vi "Ref_Num_Calibrate_Short.vi"(2 "Test Failed":refnum<vi>, 3 "Calibration Short Successful":refnum<vi>, 7 "LowCapMode?":refnum<vi>, 8 "error in":errorcluster, 9 "Keystate":string, 10 "Stop Test":refnum<vi>, 11 "Calibration Test":refnum<vi>) -> (0 "error out":errorcluster)   [LabVIEW 2020]
uses:
  <vilib>/Instr/_visa.llb/GPIB Status Boolean Array.ctl
  Global 1.vi
  <vilib>/Utility/error.llb/DialogType.ctl
panel:
  in  "error in 2":errorcluster
  out "LowCapMode?":bool
  out "message":string=" INSTRUCTIONS:\r\rNormal Use:  When using subVIs that incorporate the error in/error out (or error I/O) structure, place this handler where you want to inform the user of an error, typically at the end of the I/O data path, as the last action of the program.  If the error in error? is ERROR, the handler creates a message describing the error and its source.  If the type of dialog = 1 (default), the message is displayed to the user, who can only acknowedge it.  If the type = 2, the user can acknowledge the message or abort execution; aborting a program with active I/O is not recommended.  If the type = 0, no message is displayed; this is used to process the error programmatically, and the error out cluster elements are wired to individual terminals for that reason.  \r\rOther Use:\n\r\nlocal testing.  To test the error code of a subVI or function that does not have the error I/O structure, you can wire its error code and a source string to the local error code and error source inputs.  If error in error? indicates no error and error code is not equal to 0, the local code and source are substituted for the error in values, and error? is set TRUE (ERROR)."
  out "serial poll byte (Test 2)":i16
  out "serial poll byte (Test 1)":i16
  out "ibsta":T1
  in  "Cal_Step_Delay":u16
  out "Test Count":i32
  out "Failed Test Count":i32
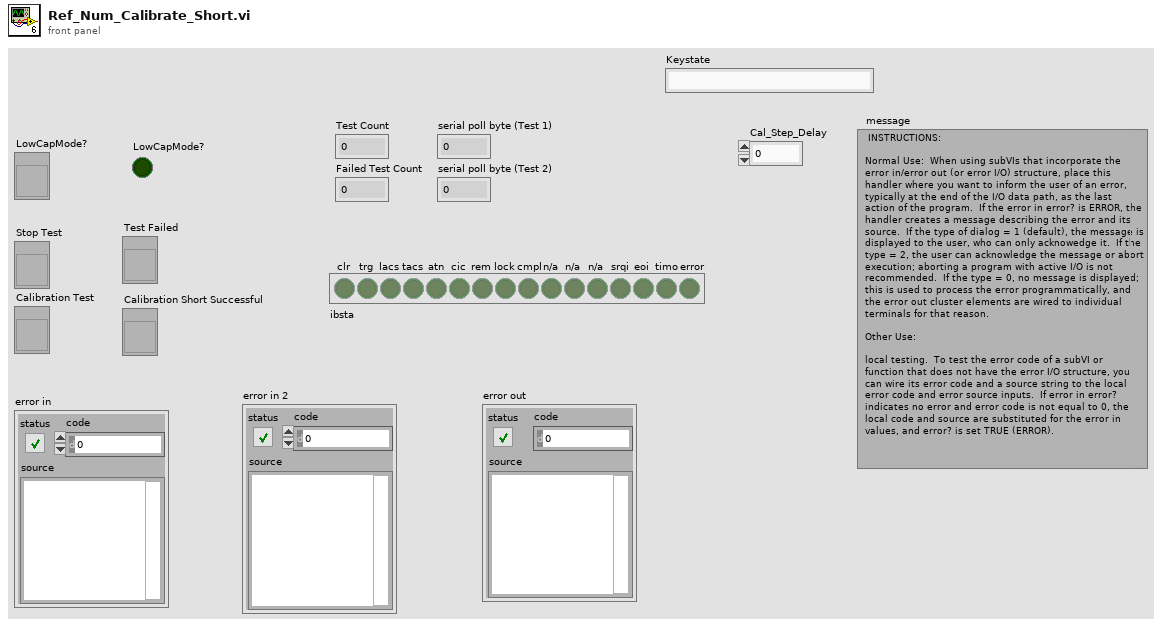
[diagram p1: front panel]
types:
  T1 = typedef "GPIB Status Boolean Array.ctl" = bool[]
  T2 = typedef "DialogType.ctl" = u16
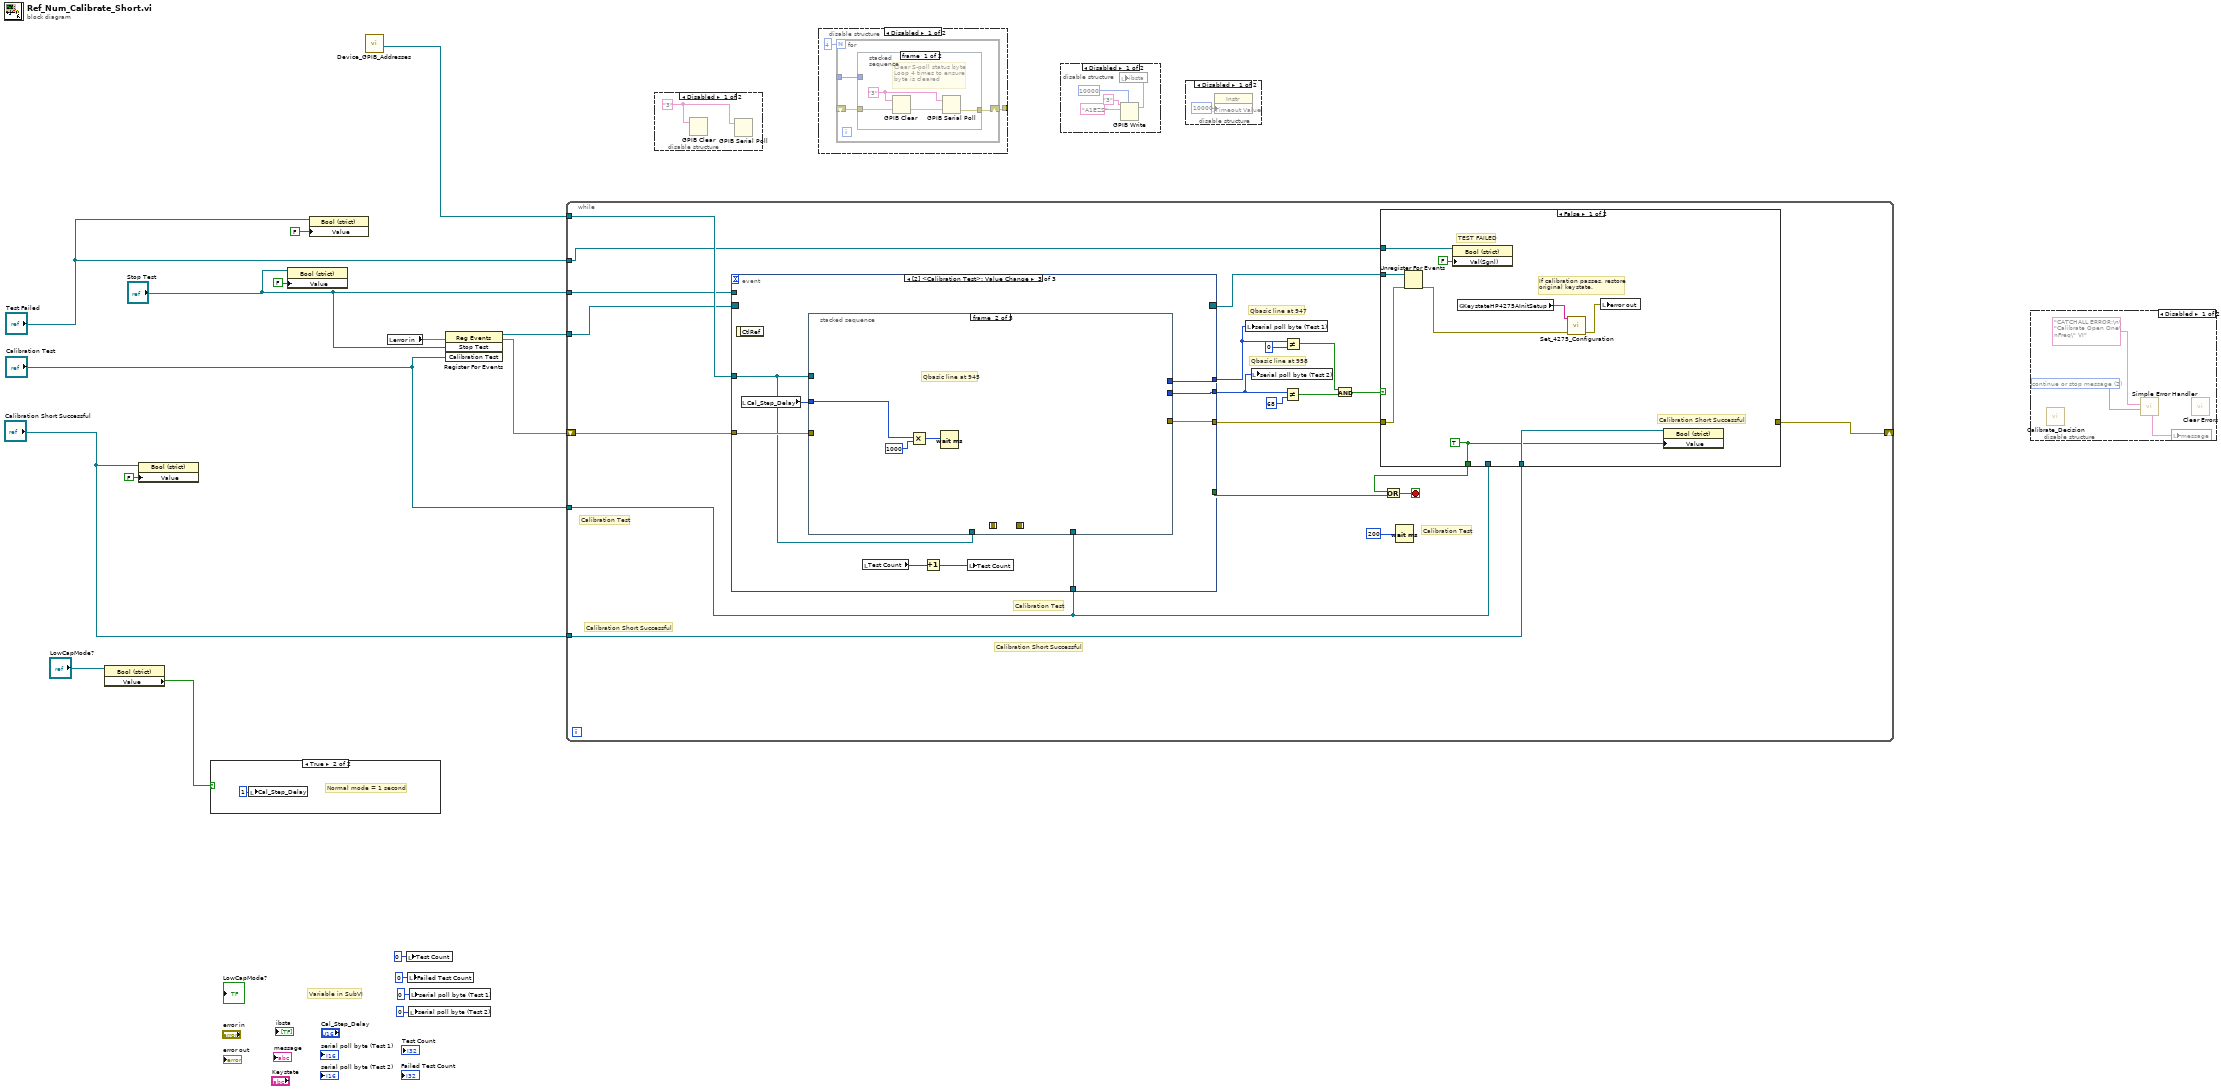
[diagram p0: block diagram]
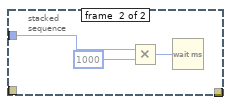
[diagram p6: hidden frame]
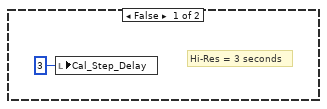
[diagram p8: hidden frame]
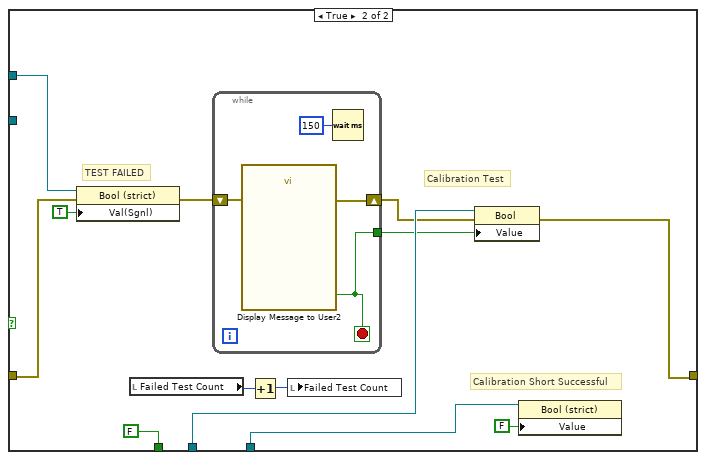
[diagram p9: hidden frame]
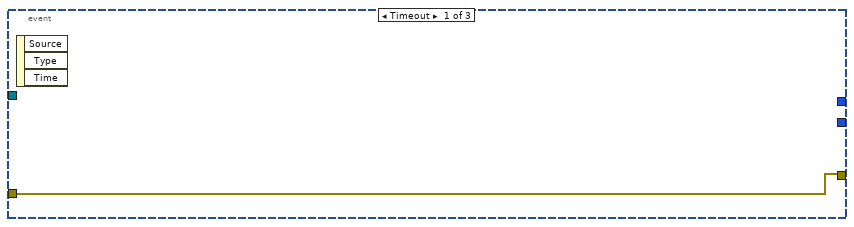
[diagram p10: hidden frame]
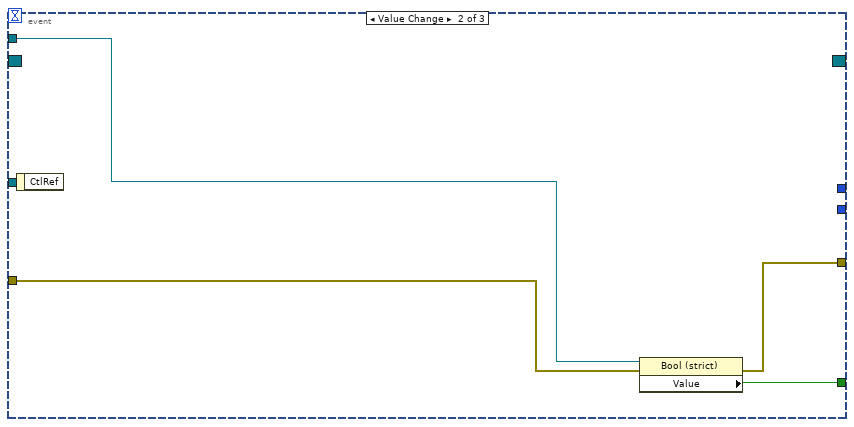
[diagram p11: hidden frame]
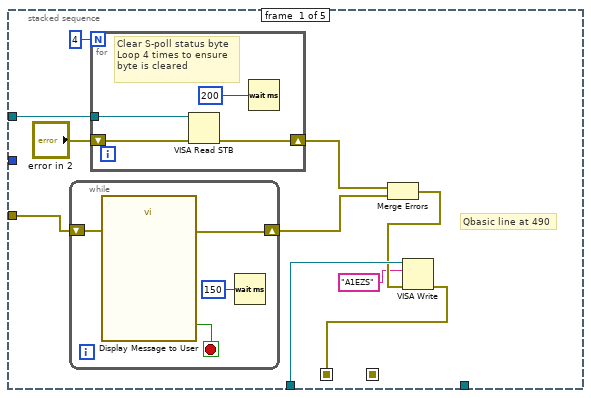
[diagram p12: hidden frame]
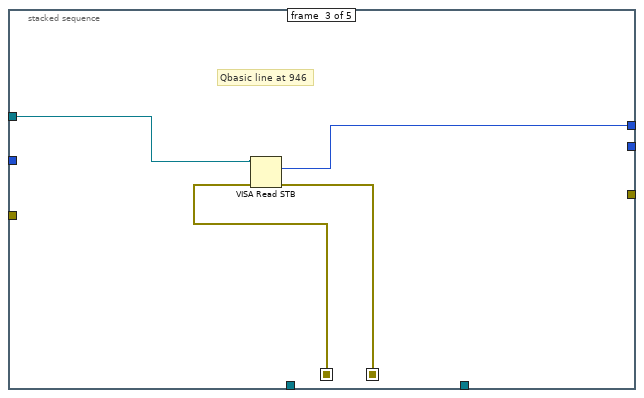
[diagram p13: hidden frame]
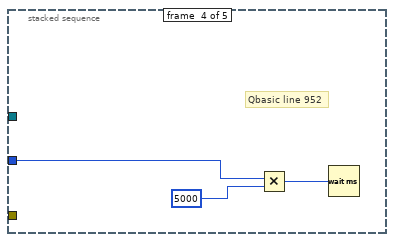
[diagram p14: hidden frame]
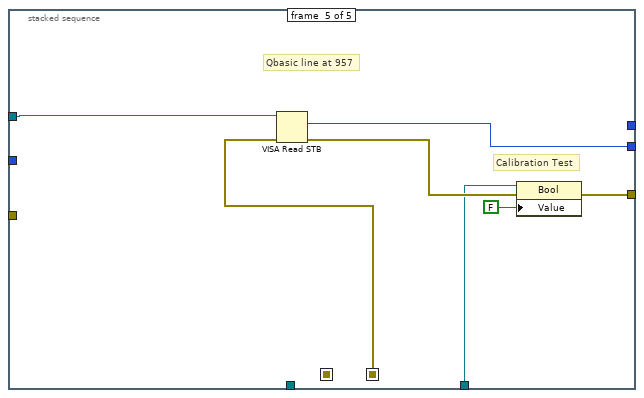
[diagram p15: hidden frame]
diagram:
  # "Variable in SubVI"
  n1 = property class="Bool (strict)"(reference="LowCapMode?") -> ("Value"=w9:bool)  [unwired: 1 in, 2 out]
  n2 = property class="Bool (strict)"(reference="Calibration Short Successful", "Value"=FALSE) -> ()  [unwired: 1 in, 2 out]
  n3 = case shown="True" w9 {
    frame False {
      # "Hi-Res = 3 seconds"
      n4 = local write "Cal_Step_Delay"(u16 3 ("Cal_Step_Delay")) -> ()
    }
    frame True {
      # "Normal mode = 1 second"
      n5 = local write "Cal_Step_Delay"(u16 1 ("CalStepDelay")) -> ()
    }
  }
  n6 = property class="Bool (strict)"(reference="Stop Test", "Value"=FALSE) -> ()  [unwired: 1 in, 2 out]
  n7 = property class="Bool (strict)"(reference="Test Failed", "Value"=FALSE) -> ()  [unwired: 1 in, 2 out]
  n8 = call "Device_GPIB_Addresses.vi"() -> ("HP 4275A Address"=w7:refnum<visa-resource-name>)  [unwired: 9 in, 2 out]
  n9 = local read "error in"() -> (w3:errorcluster)
  n10 = local write "Test Count"(0 ("Test Count")) -> ()
  n11 = local write "Failed Test Count"(0 ("Failed Test Count")) -> ()
  n12 = local write "serial poll byte (Test 2)"(i16 0 ("serial poll byte (Test 2)")) -> ()
  n13 = local write "serial poll byte (Test 1)"(i16 0 ("serial poll byte (Test 1)")) -> ()
  n14 = register-events(error in=w3, "Stop Test", "Calibration Test") -> (reference out=w2:refnum<event-registration>, error out=w1:errorcluster)  [unwired: 1 in]
  n15 = while {
    tunnel: "Calibration Test" -> [w21]
    tunnel: "Test Failed" -> [w25]
    tunnel: "Calibration Short Successful" -> [w30]
    shift-right: [w24] -> _
    shift-left: w1 -> [w26]
    tunnel: w7 -> [w29]
    tunnel: "Stop Test" -> [w28]
    tunnel: w2 -> [w27]
    stop <- w38 stop-if-true
    # "Calibration Short Successful"
    # "Calibration Test"
    # "Calibration Short Successful"
    # "Calibration Test"
    # "Calibration Test"
    # "Qbasic line at 958"
    # "Qbasic line at 947"
    n16 = event shown="[2] <Calibration Test>: Value Change" {
      selector: w27 -> [_ _ _]
      dyn-events: [_ _ _] -> w23
      timeout: _ -> [_ _ _]
      tunnel: w26 -> [w67 w69 w77]
      tunnel: [w67 w68 w72] -> w22
      tunnel: [_ w71 _] -> w39
      tunnel: [_ _ w76] -> w33
      tunnel: [_ _ w75] -> w32
      tunnel: w29 -> [_ _ w74]
      tunnel: w28 -> [_ w70 _]
      tunnel: w21 -> [_ _ w73]
      event Timeout {
        n17 = event-data() -> ()  [unwired: 1 in, 3 out]
      }
      event Value Change {
        n18 = event-data() -> ()  [unwired: 1 in, 1 out]
        n19 = property class="Bool (strict)"(reference=w70, error in=w69) -> (error out=w68:errorcluster, "Value"=w71:bool)  [unwired: 1 out]
      }
      event Value Change {
        n20 = event-data() -> ()  [unwired: 1 in, 1 out]
        n21 = local read "Cal_Step_Delay"() -> (w80:u16)
        n22 = stacked-sequence {
          seq-local: [w81 _ _ _ _] -> [_ _ w105 _ _]
          seq-local: [_ _ w103 _ _] -> [_ _ _ _ w115]
          tunnel: w77 -> [w89 _ _ _ _]
          tunnel: w80 -> [_ w100 _ w108 _]
          tunnel: [_ _ w104 _ _] -> w76
          tunnel: [_ _ _ _ w113] -> w75
          tunnel: w74 -> [w85 _ w102 _ w114]
          tunnel: w74 -> [w84 _ _ _ _]
          tunnel: [_ _ _ _ w110] -> w72
          tunnel: w73 -> [_ _ _ _ w109]
          frame #0 {
            # "Qbasic line at 490"
            n23 = while {
              shift-right: [w96] -> w88
              shift-left: w89 -> [w97]
              stop <- w98 stop-if-true
              n24 = call "Display Message to User"("error in (no error)"=w97) -> ("error out"=w96:errorcluster, "OK"=w98:bool)  [unwired: 9 in]
              n25 = Wait (ms)(milliseconds to wait=u32 150) -> ()  [unwired: 1 out]
            }
            n26 = for {
              N: 4 -> [_]
              shift-right: [w93] -> w87
              shift-left: "error in 2" -> [w94]
              tunnel: w85 -> [w92]
              # "Clear S-poll status byte\nLoop 4 times to ensure\nbyte is cleared"
              n27 = VISA Read STB(8:w94, 11:w92) -> (0:w93:errorcluster)  [unwired: 2 out]
              n28 = Wait (ms)(milliseconds to wait=u32 200) -> ()  [unwired: 1 out]
            }
            n29 = Merge Errors(w87, w88) -> (w83:errorcluster)
            n30 = VISA Write(VISA resource name=w84, write buffer="A1EZS", error in (no error)=w83) -> (error out=w81:errorcluster)  [unwired: 2 out]
          }
          frame #1 {
            # "Qbasic line at 945"
            n31 = Multiply(x=w100, y=u32 1000 ("milliseconds to wait")) -> (x*y=w99:u32)
            n32 = Wait (ms)(milliseconds to wait=w99) -> ()  [unwired: 1 out]
          }
          frame #2 {
            # "Qbasic line at 946"
            n33 = VISA Read STB(8:w105, 11:w102) -> (0:w103:errorcluster, 2:w104:u16)  [unwired: 1 out]
          }
          frame #3 {
            # "Qbasic line 952"
            n34 = Multiply(x=w108, y=u16 5000) -> (x*y=w107:u16)
            n35 = Wait (ms)(milliseconds to wait=w107) -> ()  [unwired: 1 out]
          }
          frame #4 {
            # "Calibration Test"
            # "Qbasic line at 957"
            n36 = VISA Read STB(8:w115, 11:w114) -> (0:w111:errorcluster, 2:w113:u16)  [unwired: 1 out]
            n37 = property class="Bool"(reference=w109, error in=w111, "Value"=FALSE ("Calibration Test")) -> (error out=w110:errorcluster)  [unwired: 1 out]
          }
        }
        n38 = local read "Test Count"() -> (w79:i32)
        n39 = Increment(x=w79) -> (x+1=w78:i32)
        n40 = local write "Test Count"(w78) -> ()
      }
    }
    n41 = local write "serial poll byte (Test 1)"(w33) -> ()
    n42 = local write "serial poll byte (Test 2)"(w32) -> ()
    n43 = Not Equal?(x=w32, y=i16 68) -> (x != y?=w34:bool)
    n44 = Not Equal?(x=w33, y=i16 0) -> (x != y?=w36:bool)
    n45 = And(x=w36, y=w34) -> (x .and. y?=w31:bool)
    n46 = case shown="False" w31 {
      tunnel: [w48 FALSE] -> w40
      tunnel: w22 -> [w44 w57]
      tunnel: [_ w52] -> w24
      tunnel: w30 -> [w49 w51]
      tunnel: w21 -> [_ w55]
      tunnel: w25 -> [w41 w59]
      tunnel: w23 -> [w45 _]
      frame False {
        w48 = TRUE ("Calibration Short Successful")
        # "Calibration Short Successful"
        # "TEST FAILED"
        # "If calibration passes, restore\noriginal keystate."
        n47 = Unregister For Events(event registration refnum=w45, error in=w44) -> (error out=w43:errorcluster)
        n48 = property class="Bool (strict)"(reference=w41, "Val(Sgnl)"=FALSE ("Value (Signaling)")) -> ()  [unwired: 1 in, 2 out]
        n49 = global read "Global 1.vi" "KeystateHP4275AInitSetup"() -> (w47:string)
        n50 = call "Set_4275_Configuration.vi"("error in"=w43, "Keystate"=w47) -> ("error out"=w46:errorcluster)  [unwired: 9 in]
        n51 = local write "error out"(w46) -> ()
        n52 = property class="Bool (strict)"(reference=w49, "Value"=w48) -> ()  [unwired: 1 in, 2 out]
      }
      frame True {
        # "Calibration Short Successful"
        # "Calibration Test"
        # "TEST FAILED"
        n53 = property class="Bool (strict)"(reference=w59, error in=w57, "Val(Sgnl)"=TRUE ("Value (Signaling)")) -> (error out=w56:errorcluster)  [unwired: 1 out]
        n54 = local read "Failed Test Count"() -> (w61:i32)
        n55 = while {
          tunnel: [w64] -> w54
          shift-right: [w65] -> w53
          shift-left: w56 -> [w66]
          stop <- w64 stop-if-true
          n56 = call "Display Message to User2"("error in (no error)"=w66) -> ("error out"=w65:errorcluster, "OK"=w64:bool)  [unwired: 9 in]
          n57 = Wait (ms)(milliseconds to wait=u32 150) -> ()  [unwired: 1 out]
        }
        n58 = Increment(x=w61) -> (x+1=w60:i32)
        n59 = local write "Failed Test Count"(w60) -> ()
        n60 = property class="Bool"(reference=w55, error in=w53, "Value"=w54) -> (error out=w52:errorcluster)  [unwired: 1 out]
        n61 = property class="Bool (strict)"(reference=w51, "Value"=FALSE) -> ()  [unwired: 1 in, 2 out]
      }
    }
    n62 = Or(x=w40, y=w39) -> (x .or. y?=w38:bool)
    n63 = Wait (ms)(milliseconds to wait=u32 200) -> ()  [unwired: 1 out]
  }
  n64 = disable-structure shown="Disabled" {
    frame Disabled {
      w116 = "3" ("address string")
      n65 = GPIB Clear(3:w116) -> ()  [unwired: 1 in, 2 out]
      n66 = GPIB Serial Poll(0:w116) -> ()  [unwired: 1 in, 3 out]
    }
    frame Enabled {
    }
  }
  n67 = disable-structure shown="Disabled" {
    disable-tunnel: [w117 _] -> _
    frame Disabled {
      n68 = for {
        N: 4 -> [_]
        tunnel: [w122] -> w119
        shift-right: [w121] -> w117
        shift-left: [w123] -> w120
        n69 = stacked-sequence {
          tunnel: w123 -> [w126 _]
          tunnel: w122 -> [_ w129]
          tunnel: [w127 _] -> w121
          frame #0 {
            w125 = "3" ("address string")
            # "Clear S-poll status byte\nLoop 4 times to ensure\nbyte is cleared"
            n70 = GPIB Clear(2:w126, 3:w125) -> (0:w124:errorcluster)  [unwired: 1 out]
            n71 = GPIB Serial Poll(0:w125, 1:w124) -> (4:w127:errorcluster)  [unwired: 2 out]
          }
          frame #1 {
            n72 = Multiply(x=w129, y=u32 1000 ("milliseconds to wait")) -> (x*y=w128:u32)
            n73 = Wait (ms)(milliseconds to wait=w128) -> ()  [unwired: 1 out]
          }
        }
      }
    }
    frame Enabled {
    }
  }
  n74 = disable-structure shown="Disabled" {
    frame Disabled {
      n75 = GPIB Write(0:"3" ("address string"), 1:"A1EZS" ("data"), 4:10000 ("timeout ms (488.2 global)")) -> (5:w131:bool[])  [unwired: 2 in, 1 out]
      n76 = local write "ibsta"(w131) -> ()
    }
    frame Enabled {
    }
  }
  n77 = disable-structure shown="Disabled" {
    frame Disabled {
      n78 = property class="Instr"("General Settings:Timeout Value"=u32 10000) -> ()  [unwired: 2 in, 2 out]
    }
    frame Enabled {
    }
  }
  n79 = disable-structure shown="Disabled" {
    frame Disabled {
      w137 = T2 2 items=["no dialog", "OK message", "continue or stop message", "OK message + warnings", "continue/stop + warnings"] ("type of dialog (OK msg:1)")
      n80 = call "Calibrate_Decision.vi"() -> ()  [unwired: 11 in, 1 out]
      n81 = call <vilib>:"Simple Error Handler.vi"("error source (\" \")"="CATCHALL ERROR:\n\"Calibrate Open One\nFreq\" VI" ("error source (\" \")"), "type of dialog (OK msg:1)"=w137) -> ("message"=w136:string)  [unwired: 3 in, 4 out]
      n82 = local write "message"(w136) -> ()
      n83 = call <vilib>:"Clear Errors.vi"() -> ()  [unwired: 6 in, 2 out]
    }
    frame Enabled {
    }
  }
